vi "exceptions dialog.vi"(9 "exception":T1 {"code" format="%.0x"}) -> ()   [LabVIEW 2013]
uses:
  dialog tree/VariantXControl__VP.xctl
  exception.ctl
  context.ctl
  <vilib>/addons/JSON API/Variant JSON/Variant JSON.lvlib
  <vilib>/addons/JSON API/JSON Value/JSON Value.lvclass
  exception.lvlib
panel:
  out "Variant Tree":variant(xcontrol)
  in  "copy to clipboard":bool
  in  "create report":bool
  in  "OK":bool
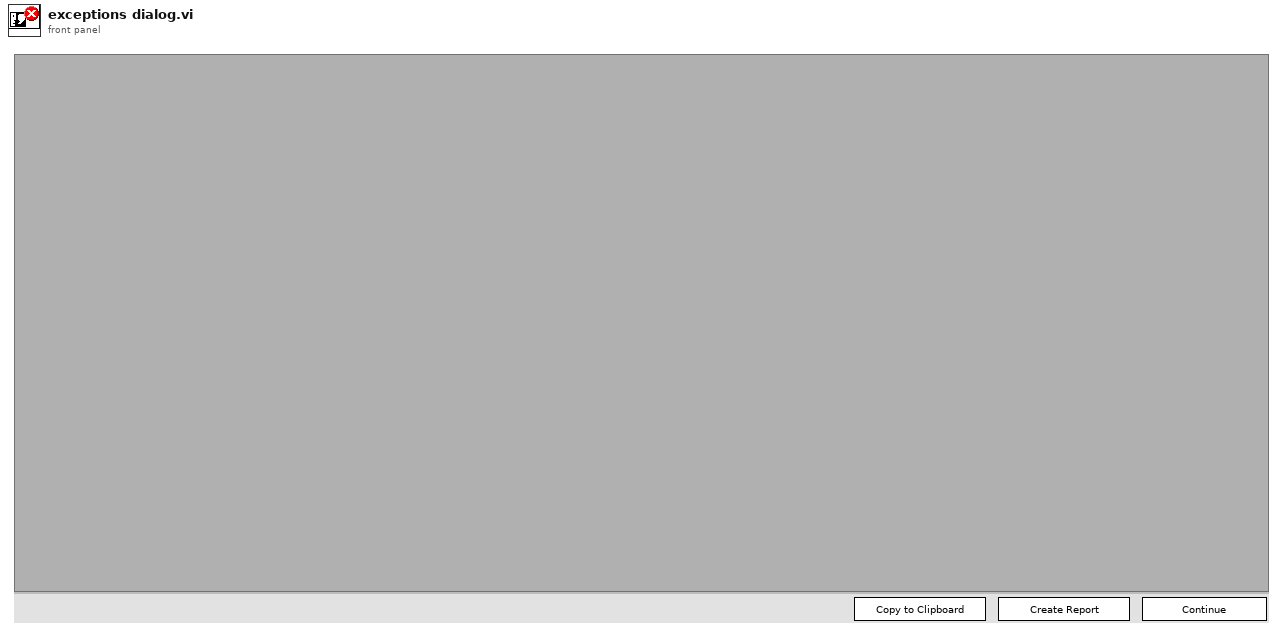
[diagram p1: front panel]
types:
  T1 = typedef "exception.lvlib/exception.ctl" = cluster{"code":i32, "context":T2, "properties":variant}
  T2 = typedef "exception.lvlib/context.ctl" = enum16{"developer", "user interface", "standard", "limited", "deterministic"}
  T3 = enum16{"open", "replace", "create", "open or create", "replace or create", "replace or create with confirmation"}
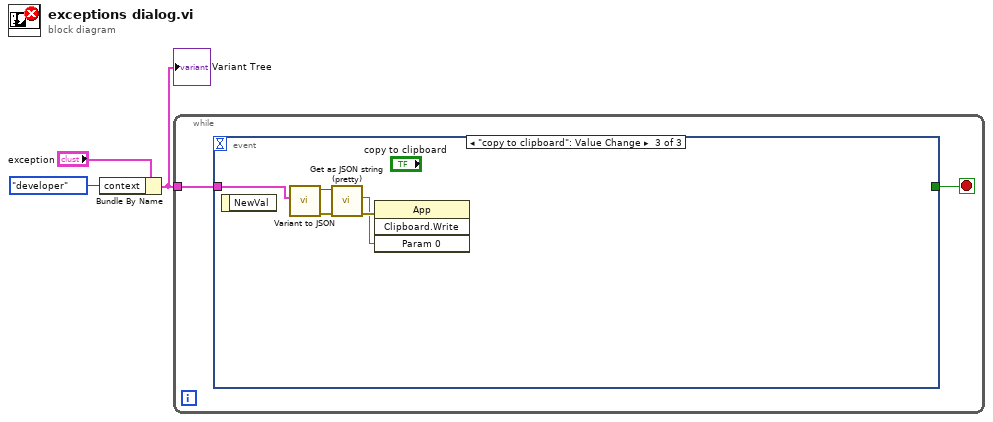
[diagram p0: block diagram]
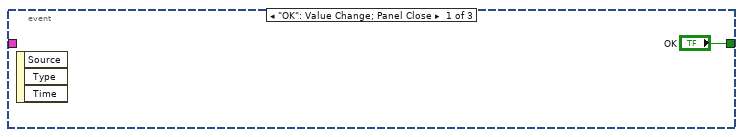
[diagram p2: hidden frame]
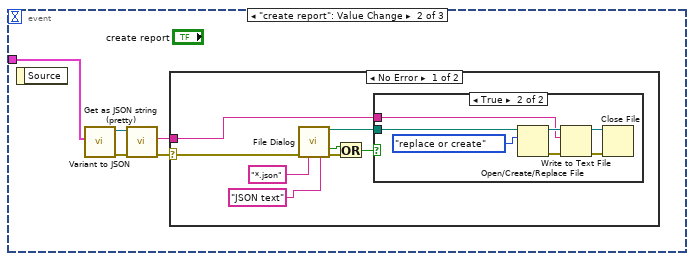
[diagram p3: hidden frame]
diagram:
  n1 = Bundle By Name(cluster="exception", "context"=context."developer") -> (w2:T1)
  "Variant Tree" <- w2
  n2 = while {
    tunnel: w2 -> [w4]
    stop <- w5 stop-if-true
    n3 = event shown="[2] \"copy to clipboard\": Value Change" {
      selector: _ -> [_ _ _]
      dyn-events: _ -> [_ _ _]
      timeout: _ -> [_ _ _]
      tunnel: ["OK" _ _] -> w5
      tunnel: w4 -> [_ w10 w27]
      event "OK": Value Change; Panel Close {
        n4 = event-data() -> ()  [unwired: 1 in, 3 out]
      }
      event "create report": Value Change {
        n5 = event-data() -> ()  [unwired: 1 in, 1 out]
        n6 = call <vilib>:"Variant to JSON.vi"("Variant"=w10) -> ("error out"=w9:errorcluster, "JSON Value out"=w11:refnum<class "JSON Value.lvclass">)  [unwired: 9 in]
        n7 = call <vilib>:"Get as JSON string (pretty).vi"("error in (no error)"=w9, "JSON Value in"=w11) -> ("error out"=w8:errorcluster, "String"=w7:string)  [unwired: 8 in]
        n8 = case shown="No Error" w8 {
          selector: w8 -> [w19 _]
          tunnel: w7 -> [w13 _]
          frame No Error {
            n9 = call "File Dialog"("error in"=w19, "pattern (all files)"="*.json", "pattern label"="JSON text") -> ("selected path"=w12:path, "cancelled"=w16:bool, "error out"=w14:errorcluster)  [unwired: 9 in, 1 out]
            n10 = Or(x=w16, y=w14) -> (x .or. y?=w15:bool)
            n11 = case shown="True" w15 {
              tunnel: w13 -> [_ w22]
              tunnel: w12 -> [_ w21]
              frame False {
              }
              frame True {
                n12 = Open/Create/Replace File(file path (use dialog)=w21, operation (0:open)=T3."replace or create") -> (refnum out=w26:refnum<file>, error out=w23:errorcluster)  [unwired: 4 in, 1 out]
                n13 = Write to Text File(file (use dialog)=w26, text=w22, error in=w23) -> (refnum out=w25:refnum<file>, error out=w24:errorcluster)  [unwired: 1 in, 1 out]
                n14 = Close File(refnum=w25, error in=w24) -> ()  [unwired: 2 out]
              }
            }
          }
          frame Error {
          }
        }
      }
      event "copy to clipboard": Value Change {
        n15 = event-data() -> ()  [unwired: 1 in, 1 out]
        n16 = call <vilib>:"Variant to JSON.vi"("Variant"=w27) -> ("error out"=w30:errorcluster, "JSON Value out"=w31:refnum<class "JSON Value.lvclass">)  [unwired: 9 in]
        n17 = call <vilib>:"Get as JSON string (pretty).vi"("error in (no error)"=w30, "JSON Value in"=w31) -> ("error out"=w29:errorcluster, "String"=w28:string)  [unwired: 8 in]
        n18 = invoke class="App" method="Clipboard.Write"(error in=w29, "Param 0"=w28) -> ()  [unwired: 2 in, 4 out]
      }
    }
  }
